vi "Pre Launch Init.vi"(11 "EventRecorder In":refnum<class "EventRecorder.lvclass">) -> (0 "Error Out":errorcluster, 3 "EventRecorder Out":refnum<class "EventRecorder.lvclass">)   [LabVIEW 2019, in "EventRecorder.lvlib" / "EventRecorder.lvclass"]
uses:
  EventRecorder.lvclass
  EventRecorder.lvclass/EventRecorder.ctl
  <vilib>/NI/Event Logger Library/EventLog/Initialize_CSV.vi
  <vilib>/NI/Event Source Actor/Event Source/Event Source/Event Source.lvclass
  <vilib>/NI/Event Logger Library/EventLog/EventLog.lvclass
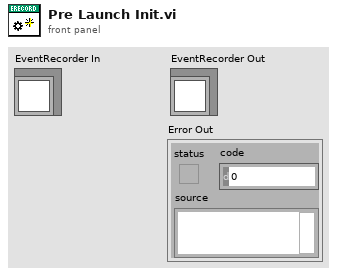
[diagram p1: front panel]
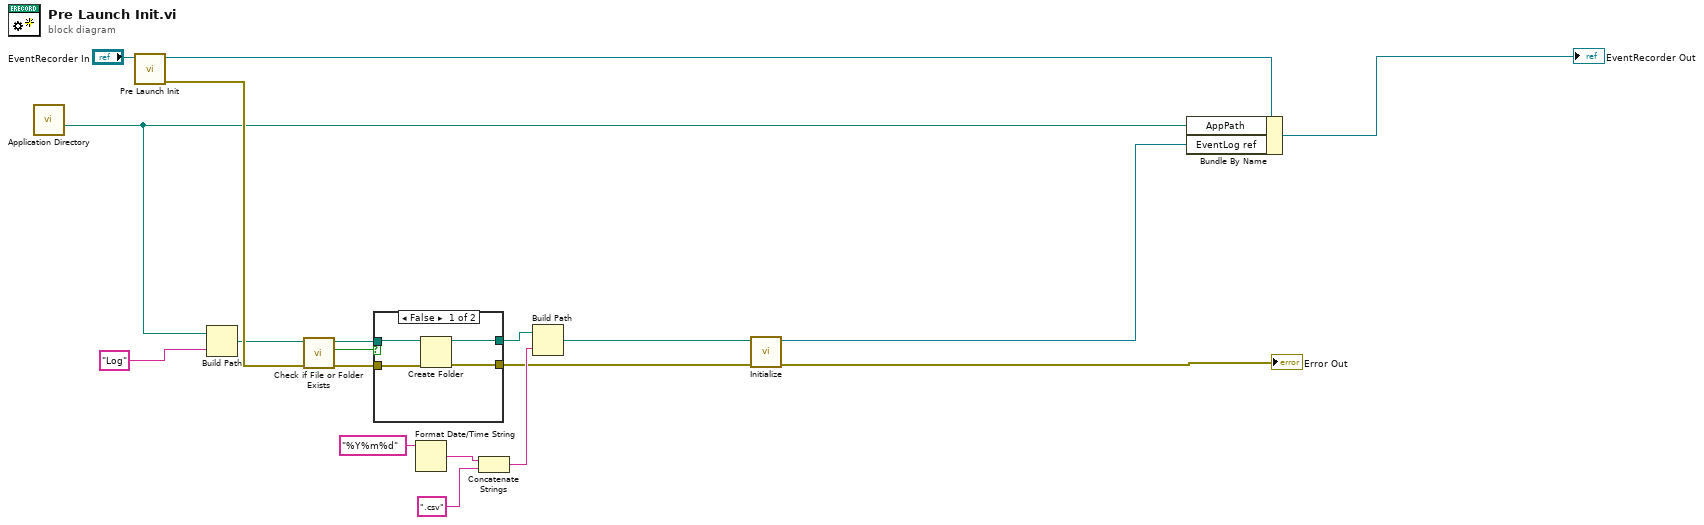
[diagram p0: block diagram]
diagram:
  n1 = call <vilib>:"Application Directory.vi"() -> ("Application Directory"=w14:path)
  n2 = call-parent "Pre Launch Init.vi"("Event Source In"="EventRecorder In") -> ("Error Out"=w16:errorcluster, "Event Source Out"=w18:refnum<class "EventRecorder.lvclass">)  [unwired: 9 in]
  n3 = Build Path(base path=w14, name or relative path="Log") -> (appended path=w8:path)
  n4 = call <vilib>:"Check if File or Folder Exists.vi"("error in (no error)"=w16, "path"=w8) -> ("error out"=w3:errorcluster, "file or folder exists?"=w7:bool, "dup path"=w6:path)  [unwired: 7 in]
  n5 = case shown="False" w7 {
    tunnel: w6 -> [w23 w25]
    tunnel: [w22 w25] -> w5
    tunnel: w3 -> [w21 w24]
    tunnel: [w20 w24] -> w1
    frame False {
      n6 = Create Folder(path (use dialog)=w23, error in=w21) -> (created path=w22:path, error out=w20:errorcluster)  [unwired: 1 in, 1 out]
    }
    frame True {
    }
  }
  n7 = Format Date/Time String(time format string (%c)="%Y%m%d") -> (date/time string=w10:string)  [unwired: 2 in]
  n8 = Concatenate Strings(w10, ".csv" ("string")) -> (w4:string)
  n9 = Build Path(base path=w5, name or relative path=w4) -> (appended path=w2:path)
  n10 = call-poly <vilib>:"Initialize.vi"("error in (no error)"=w1, "Path"=w2) -> ("error out"=→"Error Out":errorcluster, "EventLog ref"=w13:refnum<class "EventLog.lvclass">)  [unwired: 8 in]
  n11 = Bundle By Name(cluster=w18, "AppPath"=w14, "EventLog ref"=w13) -> (→"EventRecorder Out":refnum<class "EventRecorder.lvclass">)
